vi "contorno.vi"() -> ()   [LabVIEW 2020]
uses:
  <vilib>/userDefined/High Color/IMAQdx.ctl
  <vilib>/vision/Management.llb/Cast Image 2 Method.ctl
  <vilib>/vision/Contour.llb/IMAQ Connect Range Setting.ctl
  <vilib>/vision/Contour.llb/IMAQ Contour Curve Extraction.ctl
  <vilib>/vision/driver/NI_Vision_Acquisition_Software.lvlib
  <vilib>/vision/NI_Vision_Development_Module.lvlib
panel:
  in  "Session In":T1="cam1"
  in  "stop":bool
  out "Image":T2(plugin-control)
  out "Image 2":T2(plugin-control)
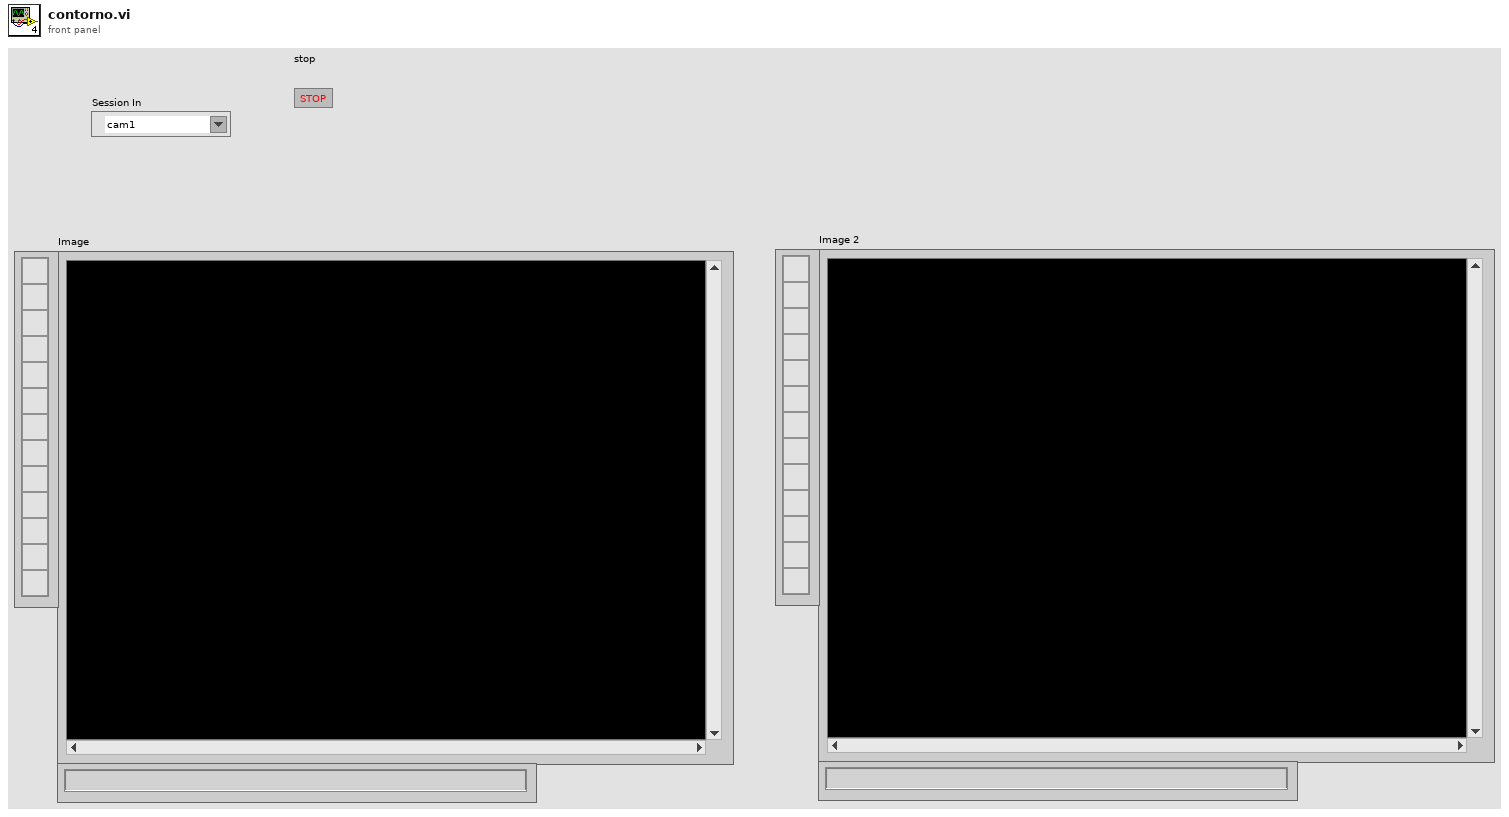
[diagram p1: front panel]
types:
  T1 = typedef "IMAQdx.ctl" = refnum<k21>
  T2 = typedef "IMAQ Image.ctl" = refnum<image>
  T3 = cluster{"Overlay?":bool, "Color":u32, "Width":u32, "Maintain Width?":bool}
  T4 = typedef "IMAQ Connect Range Setting.ctl" = cluster{"Match Constraints":u32, "Min":dbl, "Max":dbl}
  T5 = enum16{"Closest To Search Start", "Maximum Length", "Strongest Mean Gradient Change"}
  T6 = enum16{"Rect Left To Right", "Rect Right To Left", "Rect Top To Bottom", "Rect Bottom To Top", "Annulus Inner To Outer", "Annulus Outer To Inner", "Annulus Start Angle To End Angle", "Annulus End Angle To Start Angle"}
  T7 = typedef "IMAQ Contour Curve Extraction.ctl" = cluster{"Extraction Mode":u32, "Edge Threshold":i32, "Edge Filter Size":u32, "Min Length":i32, "Search Step Size":i32, "Max Endpoint Gap":i32, "Subpixel":bool}
  T8 = typedef "Image Type" = u32
  T9 = typedef "Cast Image 2 Method.ctl" = u32
  T10 = cluster{"Global Rectangle":i32[], "Contours":cluster{"Contour Type":u32, "ROI Type":u32, "Points":i32[]}[]}
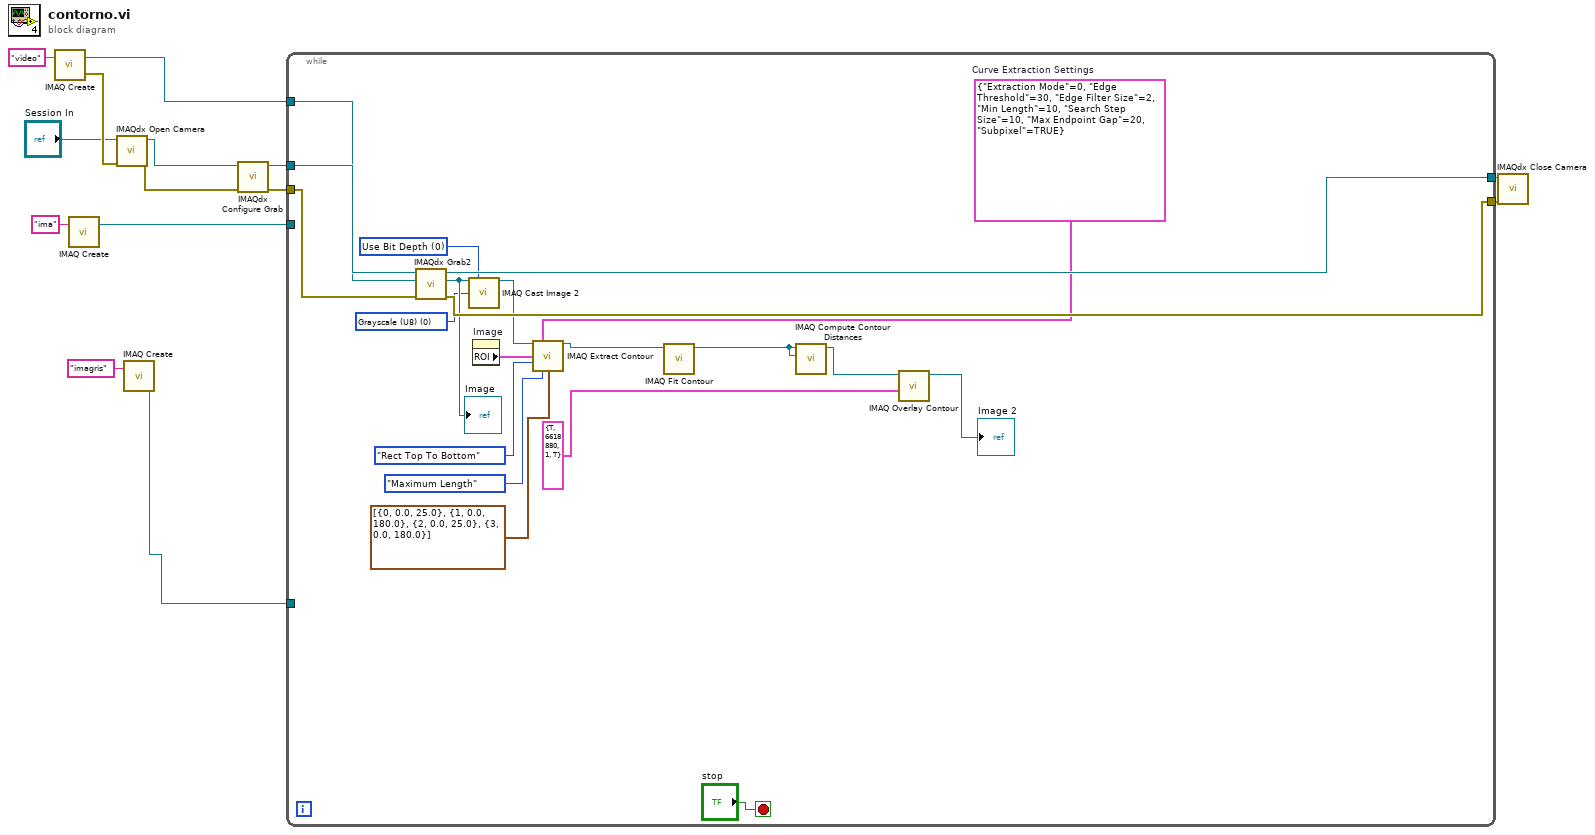
[diagram p0: block diagram]
diagram:
  n1 = call "IMAQ Create"("Image Name"="video") -> ("New Image"=w11:T2, "error out"=w14:errorcluster)  [unwired: 4 in]
  n2 = call "IMAQ Create"("Image Name"="ima") -> ("New Image"=w3:T2)  [unwired: 4 in, 1 out]
  n3 = call <vilib>:"IMAQdx Open Camera.vi"("error in"=w14, "Session In"="Session In") -> ("error out"=w7:errorcluster, "Session Out"=w13:T1)  [unwired: 8 in]
  n4 = call "IMAQ Create"("Image Name"="imagris") -> ("New Image"=w1:T2)  [unwired: 4 in, 1 out]
  n5 = call <vilib>:"IMAQdx Configure Grab.vi"("error in"=w7, "Session In"=w13) -> ("error out"=w8:errorcluster, "Session Out"=w12:T1)  [unwired: 8 in]
  n6 = while {
    tunnel: w12 -> [w34]
    tunnel: w11 -> [w33]
    tunnel: [w30] -> w10
    tunnel: [w29] -> w9
    tunnel: w8 -> [w31]
    tunnel: w3 -> [_]
    tunnel: w1 -> [_]
    stop <- "stop" stop-if-true
    w22 = T7 {"Extraction Mode"=0, "Edge Threshold"=30, "Edge Filter Size"=2, "Min Length"=10, "Search Step Size"=10, "Max Endpoint Gap"=20, "Subpixel"=TRUE}  # Curve Extraction Settings
    w26 = T8 0 items=["Grayscale (U8)", "Grayscale (I16)", "Grayscale (SGL)", "Complex (CSG)", "RGB (U32)", "HSL (U32)", "RGB (U64)", "Grayscale (U16)"] ("Image Type")
    w27 = T9 0 items=["Use Bit Depth", "Shift", "Use Lookup Table"] ("Method")
    n7 = call <vilib>:"IMAQdx Grab2.vi"("error in"=w31, "Image In"=w33, "Session In"=w34) -> ("error out"=w29:errorcluster, "Image Out"=w28:T2, "Session Out"=w30:T1)  [unwired: 5 in, 1 out]
    "Image" <- w28
    n8 = call "IMAQ Cast Image 2"("Image Src"=w28, "Method"=w27, "Image Type"=w26) -> ("Image Dst Out"=w21:T2)  [unwired: 11 in, 1 out]
    n9 = property on="Image" class="ImageControl"() -> ("ROI"=w20:T10)  [unwired: 2 in, 2 out]
    n10 = call "IMAQ Extract Contour"("Source Image"=w21, "Curve Extraction"=w22, "ROI Descriptor"=w20, "Search Direction"=T6."Rect Top To Bottom", "Contour Selection"=T5."Maximum Length", "Curve Connection"=T4[] [{"Match Constraints"=0, "Min"=0.0, "Max"=25.0}, {"Match Constraints"=1, "Min"=0.0, "Max"=180.0}, {"Match Constraints"=2, "Min"=0.0, "Max"=25.0}, {"Match Constraints"=3, "Min"=0.0, "Max"=180.0}]) -> ("Source Image Out"=w17:T2)  [unwired: 2 in, 7 out]
    n11 = call-poly "IMAQ Fit Contour"("Contour Image"=w17) -> ("Contour Image Out"=w16:T2)  [unwired: 2 in, 8 out]
    n12 = call "IMAQ Compute Contour Distances"("Template Contour Image"=w16, "Target Contour Image"=w16) -> ("Target Contour Image Out (dup)"=w15:T2)  [unwired: 3 in, 6 out]
    n13 = call "IMAQ Overlay Contour"("Contour Points Settings"=T3 {"Overlay?"=TRUE, "Color"=6618880, "Width"=1, "Maintain Width?"=TRUE}, "Image"=w15) -> ("Image Out"=→"Image 2":T2)  [unwired: 4 in, 5 out]
  }
  n14 = call <vilib>:"IMAQdx Close Camera.vi"("error in"=w9, "Session In"=w10) -> ()  [unwired: 9 in, 1 out]
